vi "Project.vi"() -> ()   [LabVIEW 2016]
uses:
  <vilib>/DAQmx/read.llb/DAQmx Read (Digital Bool 1Line 1Point).vi
  <vilib>/DAQmx/write.llb/DAQmx Write (Digital Bool 1Line 1Point).vi
  <vilib>/DAQmx/create/channels.llb/DAQmx Create Channel (DO-Digital Output).vi
  <vilib>/DAQmx/create/channels.llb/DAQmx Create Channel (DI-Digital Input).vi
  <vilib>/DAQmx/miscellaneous.llb/DAQmx Fill In Error Info.vi
  <vilib>/ptbypt/NI_PtbyPt.lvlib
panel:
  in  "Emergency Stop":bool
  out "Use R2":bool
  out "Use R1":bool
  out "Register Bit #1":bool
  out "Register Bit #2":bool
  out "Output Queue Counter":dbl
  out "Rejection Pusher":bool
  out "Metal Sensor 2":bool
  out "Proximity Sensor":bool
  out "Complete or not":bool
  out "Plastic In Queue":dbl
  out "Hopper":bool
  out "Pusher":bool=TRUE
  out "Plastic or not":bool
  out "Belt 2":bool=TRUE
  out "Belt 1":bool=TRUE
  out "Stoped":bool=TRUE
  out "Started":bool=TRUE
  in  "PAUSE":bool
  in  "OFF":bool
  in  "ON":bool
  out "Rejected Pieces":dbl
  out "Completed Pieces":dbl
  out "Don't Push?":bool
  out "Is there anything there?":bool
  # "Main Control"
  # "Sorting Station"
  # "QA Sorting Station"
  # "QA Sorting Register Value"
  # "Result Counter"
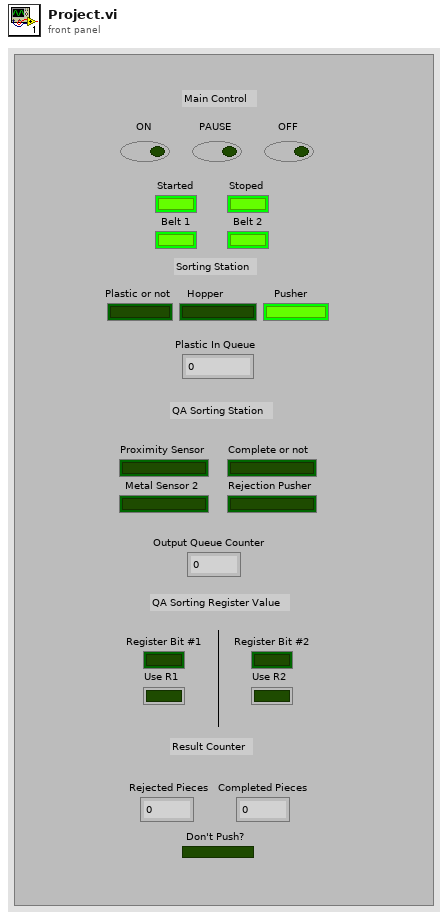
[diagram p1: front panel]
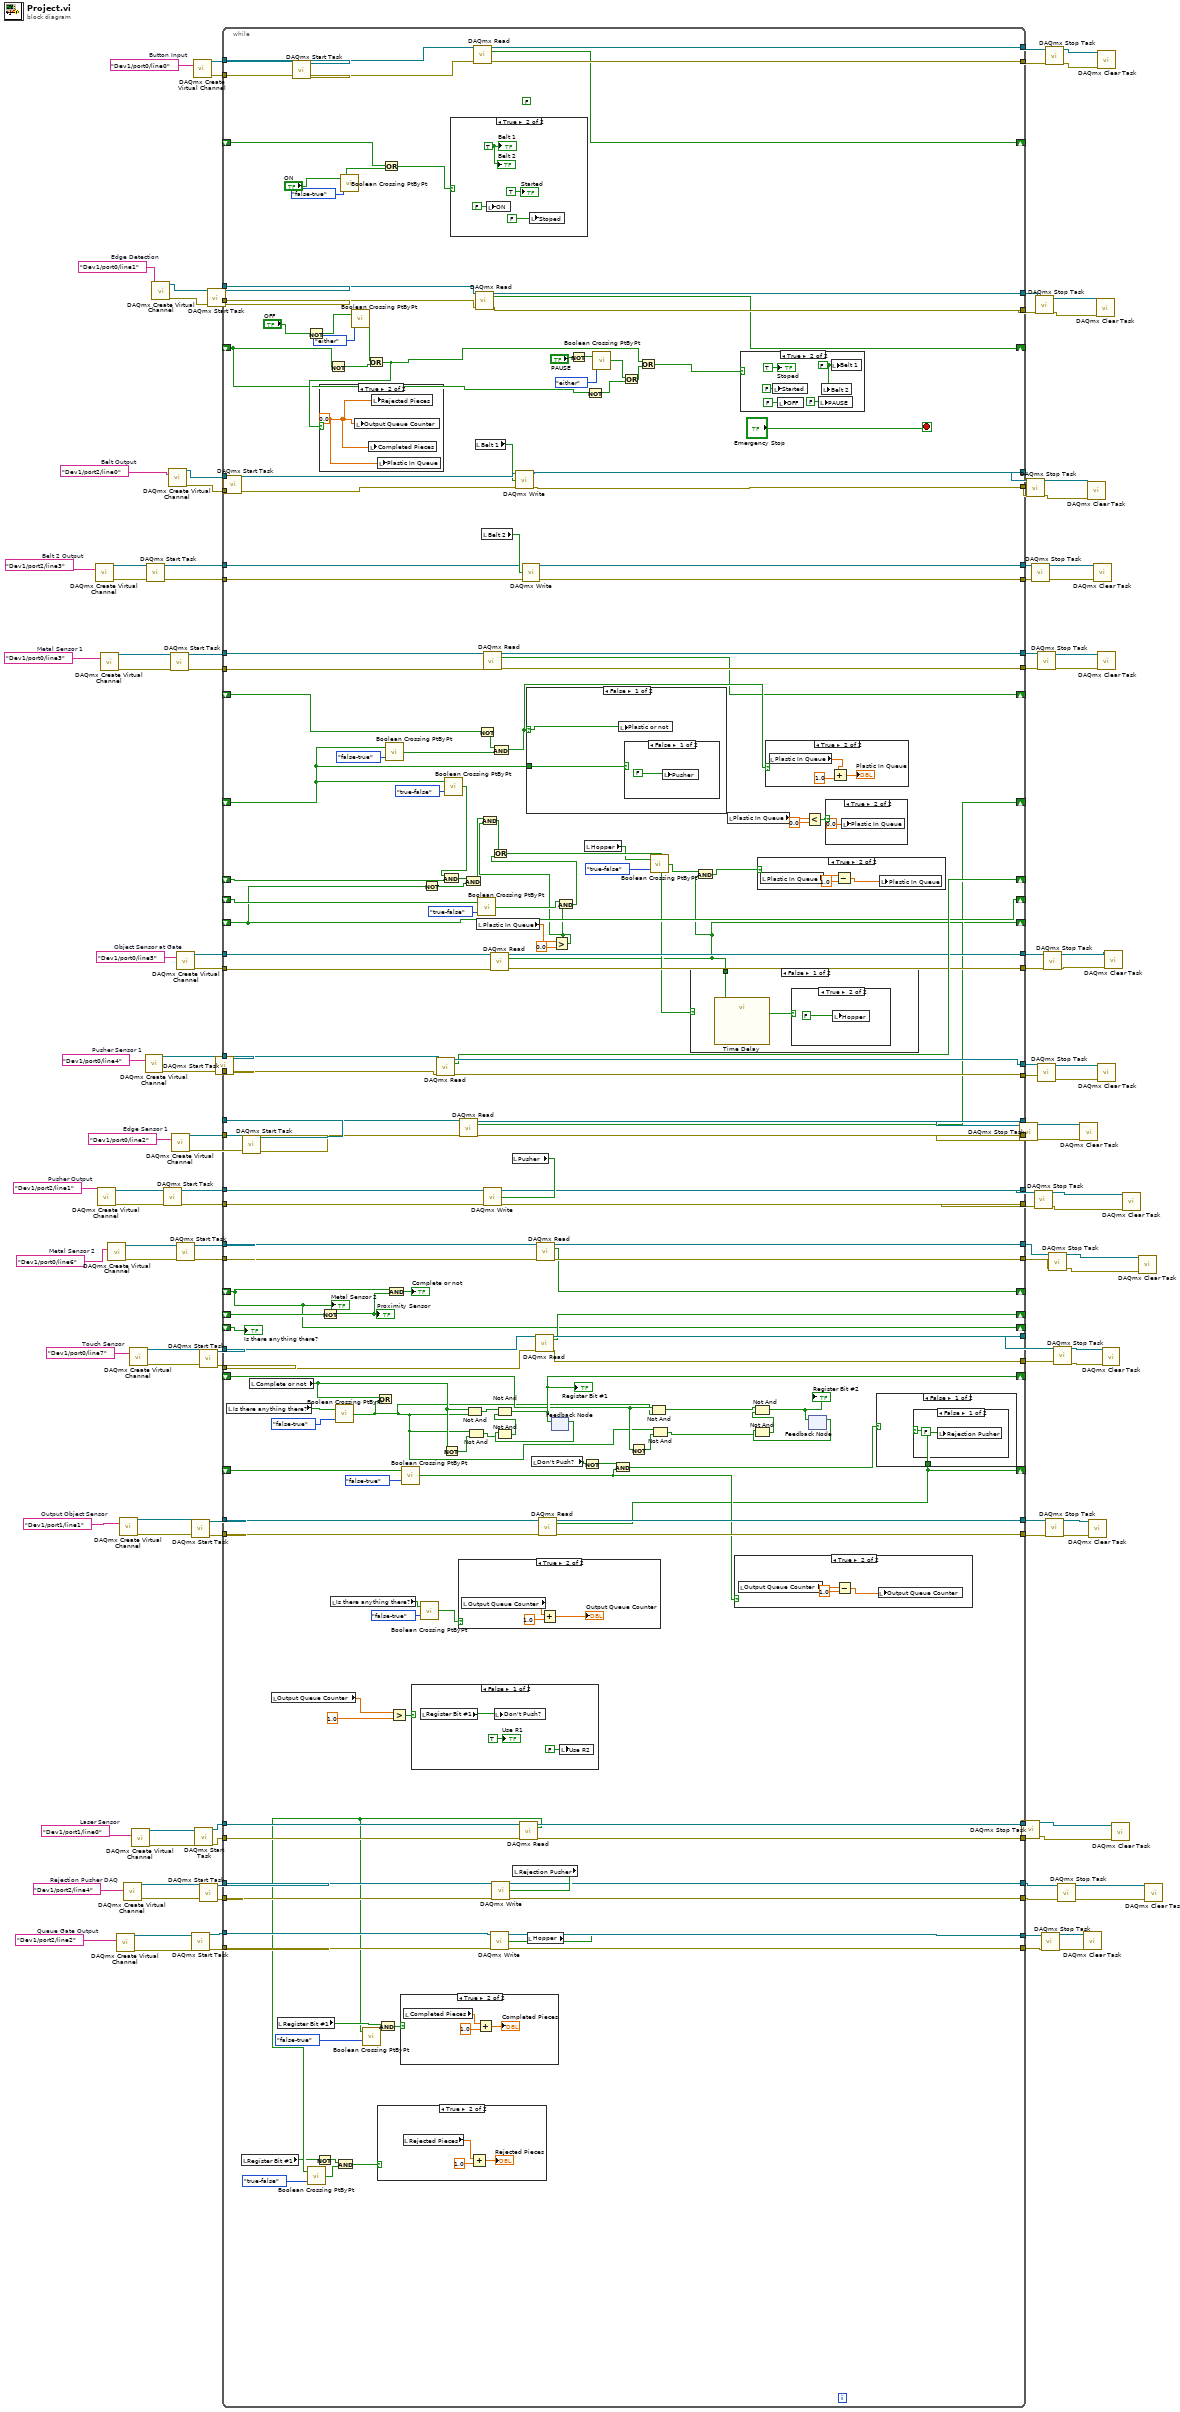
[diagram p0: block diagram]
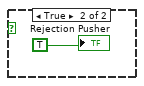
[diagram p3: hidden frame]
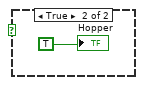
[diagram p5: hidden frame]
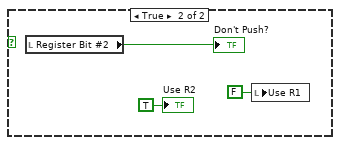
[diagram p12: hidden frame]
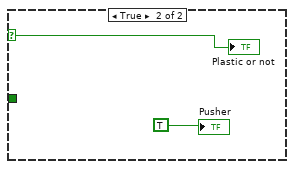
[diagram p16: hidden frame]
diagram:
  w5 = tag "Dev1/port0/line5"  # Object Sensor at Gate
  w12 = tag "Dev1/port1/line0"  # Laser Sensor
  w25 = tag "Dev1/port0/line7"  # Touch Sensor
  w28 = tag "Dev1/port1/line1"  # Output Object Sensor
  w43 = tag "Dev1/port0/line6"  # Metal Sensor 2
  w46 = tag "Dev1/port2/line4"  # Rejection Pusher DAQ
  w57 = tag "Dev1/port2/line2"  # Queue Gate Output
  w64 = tag "Dev1/port2/line3"  # Belt 2 Output
  w75 = tag "Dev1/port0/line4"  # Pusher Sensor 1
  w84 = tag "Dev1/port0/line2"  # Edge Sensor 1
  w89 = tag "Dev1/port2/line1"  # Pusher Output
  w90 = tag "Dev1/port0/line1"  # Edge Detection
  w91 = tag "Dev1/port0/line0"  # Button Input
  w92 = tag "Dev1/port0/line3"  # Metal Sensor 1
  w93 = tag "Dev1/port2/line0"  # Belt Output
  n1 = call-poly <vilib>:"DAQmx Create Virtual Channel.vi"("lines"=w64) -> ("task out"=w66:refnum<k21>, "error out"=w65:errorcluster)  [unwired: 13 in]
  n2 = call-poly <vilib>:"DAQmx Create Virtual Channel.vi"("lines"=w89) -> ("task out"=w101:refnum<k21>, "error out"=w100:errorcluster)  [unwired: 13 in]
  n3 = call-poly <vilib>:"DAQmx Create Virtual Channel.vi"("lines"=w92) -> ("task out"=w109:refnum<k21>, "error out"=w108:errorcluster)  [unwired: 13 in]
  n4 = call-poly <vilib>:"DAQmx Create Virtual Channel.vi"("lines"=w43) -> ("task out"=w45:refnum<k21>, "error out"=w44:errorcluster)  [unwired: 13 in]
  n5 = call-poly <vilib>:"DAQmx Create Virtual Channel.vi"("lines"=w57) -> ("task out"=w59:refnum<k21>, "error out"=w58:errorcluster)  [unwired: 13 in]
  n6 = call-poly <vilib>:"DAQmx Create Virtual Channel.vi"("lines"=w28) -> ("task out"=w30:refnum<k21>, "error out"=w29:errorcluster)  [unwired: 13 in]
  n7 = call-poly <vilib>:"DAQmx Create Virtual Channel.vi"("lines"=w46) -> ("task out"=w48:refnum<k21>, "error out"=w47:errorcluster)  [unwired: 13 in]
  n8 = call-poly <vilib>:"DAQmx Create Virtual Channel.vi"("lines"=w25) -> ("task out"=w27:refnum<k21>, "error out"=w26:errorcluster)  [unwired: 13 in]
  n9 = call-poly <vilib>:"DAQmx Create Virtual Channel.vi"("lines"=w12) -> ("task out"=w14:refnum<k21>, "error out"=w13:errorcluster)  [unwired: 13 in]
  n10 = call-poly <vilib>:"DAQmx Create Virtual Channel.vi"("lines"=w75) -> ("task out"=w77:refnum<k21>, "error out"=w76:errorcluster)  [unwired: 13 in]
  n11 = call <vilib>:"DAQmx Start Task.vi"("task/channels in"=w66, "error in"=w65) -> ("task out"=w63:refnum<k21>, "error out"=w62:errorcluster)  [unwired: 12 in]
  n12 = call-poly <vilib>:"DAQmx Create Virtual Channel.vi"("lines"=w90) -> ("task out"=w125:refnum<k21>, "error out"=w124:errorcluster)  [unwired: 13 in]
  n13 = call <vilib>:"DAQmx Start Task.vi"("task/channels in"=w101, "error in"=w100) -> ("task out"=w95:refnum<k21>, "error out"=w94:errorcluster)  [unwired: 12 in]
  n14 = call-poly <vilib>:"DAQmx Create Virtual Channel.vi"("lines"=w93) -> ("task out"=w113:refnum<k21>, "error out"=w112:errorcluster)  [unwired: 13 in]
  n15 = call <vilib>:"DAQmx Start Task.vi"("task/channels in"=w109, "error in"=w108) -> ("task out"=w107:refnum<k21>, "error out"=w106:errorcluster)  [unwired: 12 in]
  n16 = call-poly <vilib>:"DAQmx Create Virtual Channel.vi"("lines"=w84) -> ("task out"=w86:refnum<k21>, "error out"=w85:errorcluster)  [unwired: 13 in]
  n17 = call <vilib>:"DAQmx Start Task.vi"("task/channels in"=w45, "error in"=w44) -> ("task out"=w40:refnum<k21>, "error out"=w39:errorcluster)  [unwired: 12 in]
  n18 = call-poly <vilib>:"DAQmx Create Virtual Channel.vi"("lines"=w5) -> ("task out"=w4:refnum<k21>, "error out"=w3:errorcluster)  [unwired: 13 in]
  n19 = call <vilib>:"DAQmx Start Task.vi"("task/channels in"=w30, "error in"=w29) -> ("task out"=w24:refnum<k21>, "error out"=w23:errorcluster)  [unwired: 12 in]
  n20 = call <vilib>:"DAQmx Start Task.vi"("task/channels in"=w59, "error in"=w58) -> ("task out"=w56:refnum<k21>, "error out"=w55:errorcluster)  [unwired: 12 in]
  n21 = call-poly <vilib>:"DAQmx Create Virtual Channel.vi"("lines"=w91) -> ("task out"=w133:refnum<k21>, "error out"=w132:errorcluster)  [unwired: 13 in]
  n22 = call <vilib>:"DAQmx Start Task.vi"("task/channels in"=w14, "error in"=w13) -> ("task out"=w11:refnum<k21>, "error out"=w8:errorcluster)  [unwired: 12 in]
  n23 = call <vilib>:"DAQmx Start Task.vi"("task/channels in"=w27, "error in"=w26) -> ("task out"=w22:refnum<k21>, "error out"=w21:errorcluster)  [unwired: 12 in]
  n24 = call <vilib>:"DAQmx Start Task.vi"("task/channels in"=w48, "error in"=w47) -> ("task out"=w38:refnum<k21>, "error out"=w37:errorcluster)  [unwired: 12 in]
  n25 = call <vilib>:"DAQmx Start Task.vi"("task/channels in"=w125, "error in"=w124) -> ("task out"=w122:refnum<k21>, "error out"=w123:errorcluster)  [unwired: 12 in]
  n26 = call <vilib>:"DAQmx Start Task.vi"("task/channels in"=w77, "error in"=w76) -> ("task out"=w74:refnum<k21>, "error out"=w73:errorcluster)  [unwired: 12 in]
  n27 = call <vilib>:"DAQmx Start Task.vi"("task/channels in"=w113, "error in"=w112) -> ("task out"=w111:refnum<k21>, "error out"=w110:errorcluster)  [unwired: 12 in]
  n28 = call <vilib>:"DAQmx Start Task.vi"("task/channels in"=w86, "error in"=w85) -> ("task out"=w83:refnum<k21>, "error out"=w82:errorcluster)  [unwired: 12 in]
  n29 = call <vilib>:"DAQmx Start Task.vi"("task/channels in"=w133, "error in"=w132) -> ("task out"=w131:refnum<k21>, "error out"=w130:errorcluster)  [unwired: 12 in]
  n30 = while {
    tunnel: w131 -> [w300]
    tunnel: w130 -> [w299]
    tunnel: [w298] -> w129
    tunnel: [w297] -> w128
    shift-right: [w295] -> _
    shift-left: _ -> [w229]
    tunnel: w123 -> [w294]
    tunnel: w122 -> [w293]
    tunnel: [w292] -> w121
    tunnel: [w291] -> w118
    shift-right: [w290] -> _
    shift-left: _ -> [w167]
    tunnel: [w289] -> w115
    tunnel: [w286] -> w114
    tunnel: w111 -> [w288]
    tunnel: w110 -> [w287]
    tunnel: w107 -> [w284]
    tunnel: w106 -> [w283]
    tunnel: [w282] -> w103
    tunnel: [w281] -> w102
    shift-right: [w139] -> _
    shift-left: _ -> [w138]
    tunnel: [w279] -> w97
    tunnel: [w278] -> w96
    tunnel: w95 -> [w277]
    tunnel: w94 -> [w276]
    tunnel: w83 -> [w275]
    tunnel: w82 -> [w274]
    tunnel: [w273] -> w81
    tunnel: [w272] -> w80
    shift-right: [w141] -> _
    shift-left: _ -> [w134]
    tunnel: w74 -> [w270]
    tunnel: w73 -> [w269]
    tunnel: [w268] -> w72
    tunnel: [w267] -> w71
    tunnel: [w264] -> w68
    tunnel: [w263] -> w67
    tunnel: w63 -> [w262]
    tunnel: w62 -> [w261]
    tunnel: w56 -> [w260]
    tunnel: w55 -> [w259]
    tunnel: [w258] -> w54
    tunnel: [w257] -> w53
    shift-right: [w255] -> _
    shift-left: _ -> [w254]
    tunnel: [w250] -> w42
    tunnel: [w249] -> w41
    tunnel: w40 -> [w248]
    tunnel: w39 -> [w247]
    tunnel: w38 -> [w246]
    tunnel: w37 -> [w245]
    tunnel: [w244] -> w36
    tunnel: [w243] -> w35
    shift-right: [w242] -> _
    shift-left: _ -> [w195]
    tunnel: w24 -> [w241]
    tunnel: w23 -> [w240]
    tunnel: w22 -> [w239]
    tunnel: w21 -> [w238]
    tunnel: [w237] -> w20
    tunnel: [w236] -> w19
    tunnel: [w235] -> w18
    tunnel: [w234] -> w17
    shift-right: [w142] -> _
    shift-left: _ -> [w217]
    shift-right: [w233] -> _
    shift-left: _ -> [w232]
    shift-right: [w195] -> _
    shift-left: _ -> [w219]
    tunnel: w11 -> [w215]
    tunnel: [w214] -> w10
    tunnel: [w213] -> w9
    tunnel: w8 -> [w212]
    shift-right: [w197] -> _
    shift-left: _ -> [w196]
    tunnel: w4 -> [w166]
    tunnel: w3 -> [w165]
    tunnel: [w164] -> w2
    tunnel: [w163] -> w1
    shift-right: [w136] -> _
    shift-left: _ -> [w158]
    shift-right: [w158] -> _
    shift-left: _ -> [w161]
    stop <- "Emergency Stop" stop-if-true
    (unwired) FALSE ("Boolean")
    n31 = local read "Is there anything there?"() -> (w220:bool)
    n32 = local read "Register Bit #1"() -> (w176:bool)
    n33 = local read "Complete or not"() -> (w194:bool)
    n34 = local read "Output Queue Counter"() -> (w205:dbl)
    n35 = local read "Register Bit #1"() -> (w183:bool)
    n36 = Not(x="OFF") -> (.not. x?=w189:bool)
    n37 = Not(x=w176) -> (.not. x?=w177:bool)
    n38 = Not(x=w232) -> (.not. x?=w227:bool)
    "Proximity Sensor" <- w227
    n39 = Not(x=w167) -> (.not. x?=w228:bool)
    n40 = local read "Is there anything there?"() -> (w209:bool)
    n41 = call <vilib>:"Boolean Crossing PtByPt.vi"("direction"=enum16{"either", "false-true", "true-false"}."false-true", "input"=w220) -> ("crossing"=w193:bool)  [unwired: 1 in]
    n42 = call <vilib>:"Boolean Crossing PtByPt.vi"("direction"=enum16{"either", "false-true", "true-false"}."false-true", "input"="ON") -> ("crossing"=w192:bool)  [unwired: 1 in]
    n43 = call <vilib>:"Boolean Crossing PtByPt.vi"("direction"=enum16{"either", "false-true", "true-false"}."either", "input"=w189) -> ("crossing"=w190:bool)  [unwired: 1 in]
    n44 = Or(x=w190, y=w228) -> (x .or. y?=w168:bool)
    n45 = case shown="True" w168 {
      frame False {
      }
      frame True {
        w314 = 0.0 ("Completed Piece")
        n46 = local write "Output Queue Counter"(w314) -> ()
        n47 = local write "Completed Pieces"(w314) -> ()
        n48 = local write "Rejected Pieces"(w314) -> ()
        n49 = local write "Plastic In Queue"(w314) -> ()
      }
    }
    n50 = Or(x=w194, y=w193) -> ()  [unwired: 1 out]
    n51 = Or(x=w229, y=w192) -> (x .or. y?=w230:bool)
    n52 = call <vilib>:"Boolean Crossing PtByPt.vi"("direction"=enum16{"either", "false-true", "true-false"}."false-true", "input"=w134) -> ("crossing"=w256:bool)  [unwired: 1 in]
    n53 = And(x=w195, y=w227) -> (x .and. y?=→"Complete or not":bool)
    n54 = Greater?(x=w205, y=1.0) -> (0:w204:bool)
    n55 = call <vilib>:"Boolean Crossing PtByPt.vi"("direction"=enum16{"either", "false-true", "true-false"}."false-true", "input"=w217) -> ("crossing"=w207:bool)  [unwired: 1 in]
    n56 = case shown="False" w204 {
      frame False {
        n57 = local read "Register Bit #1"() -> (w323:bool)
        n58 = local write "Don't Push?"(w323) -> ()
        n59 = local write "Use R2"(FALSE ("Use R2")) -> ()
        "Use R1" <- TRUE ("Use R1")
      }
      frame True {
        n60 = local read "Register Bit #2"() -> (→"Don't Push?":bool)
        n61 = local write "Use R1"(FALSE ("Use R1")) -> ()
        "Use R2" <- TRUE ("Use R2")
      }
    }
    n62 = call <vilib>:"Boolean Crossing PtByPt.vi"("direction"=enum16{"either", "false-true", "true-false"}."false-true", "input"=w209) -> ("crossing"=w210:bool)  [unwired: 1 in]
    n63 = Not(x=w158) -> (.not. x?=w159:bool)
    n64 = call-poly <vilib>:"DAQmx Read.vi"("task/channels in"=w270, "error in"=w269) -> ("task out"=w267:refnum<k21>, "data"=w255:bool, "error out"=w268:errorcluster)  [unwired: 11 in]
    n65 = Not(x=w194) -> (.not. x?=w222:bool)
    n66 = call <vilib>:"Boolean Crossing PtByPt.vi"("direction"=enum16{"either", "false-true", "true-false"}."true-false", "input"=w134) -> ("crossing"=w252:bool)  [unwired: 1 in]
    n67 = And(x=w252, y=w254) -> (x .and. y?=w160:bool)
    n68 = case shown="True" w230 {
      frame False {
      }
      frame True {
        w344 = TRUE
        n69 = local write "ON"(FALSE ("ON")) -> ()
        n70 = local write "Stoped"(FALSE) -> ()
        "Started" <- TRUE ("Boolean")
        "Belt 1" <- w344
        "Belt 2" <- w344
      }
    }
    n71 = case shown="True" w210 {
      frame False {
      }
      frame True {
        n72 = local read "Output Queue Counter"() -> (w330:dbl)
        n73 = Add(x=w330, y=1.0) -> (x+y=→"Output Queue Counter":dbl)
      }
    }
    n74 = call-poly <vilib>:"DAQmx Read.vi"("task/channels in"=w275, "error in"=w274) -> ("task out"=w272:refnum<k21>, "data"=w141:bool, "error out"=w273:errorcluster)  [unwired: 11 in]
    n75 = And(x=w160, y=w159) -> (x .and. y?=w152:bool)
    n76 = Not And(1:w193, 2:w194) -> (0:w223:bool)
    n77 = Not And(1:w222, 2:w193) -> (0:w224:bool)
    n78 = call-poly <vilib>:"DAQmx Read.vi"("task/channels in"=w300, "error in"=w299) -> ("task out"=w298:refnum<k21>, "data"=w295:bool, "error out"=w297:errorcluster)  [unwired: 11 in]
    n79 = call-poly <vilib>:"DAQmx Read.vi"("task/channels in"=w293, "error in"=w294) -> ("task out"=w292:refnum<k21>, "data"=w290:bool, "error out"=w291:errorcluster)  [unwired: 11 in]
    n80 = local read "Belt 1"() -> (w285:bool)
    n81 = local read "Plastic In Queue"() -> (w156:dbl)
    n82 = call <vilib>:"Boolean Crossing PtByPt.vi"("direction"=enum16{"either", "false-true", "true-false"}."true-false", "input"=w161) -> ("crossing"=w154:bool)  [unwired: 1 in]
    n83 = Not(x=w138) -> (.not. x?=w271:bool)
    n84 = local read "Belt 2"() -> (w265:bool)
    n85 = call-poly <vilib>:"DAQmx Read.vi"("task/channels in"=w284, "error in"=w283) -> ("task out"=w282:refnum<k21>, "data"=w139:bool, "error out"=w281:errorcluster)  [unwired: 11 in]
    n86 = call-poly <vilib>:"DAQmx Read.vi"("task/channels in"=w166, "error in"=w165) -> ("task out"=w164:refnum<k21>, "data"=w136:bool, "error out"=w163:errorcluster)  [unwired: 11 in]
    n87 = And(x=w271, y=w256) -> (x .and. y?=w157:bool)
    n88 = local read "Pusher"() -> (w280:bool)
    n89 = call-poly <vilib>:"DAQmx Write.vi"("task/channels in"=w277, "data"=w280, "error in"=w276) -> ("task out"=w279:refnum<k21>, "error out"=w278:errorcluster)  [unwired: 10 in, 1 out]
    n90 = local read "Rejection Pusher"() -> (w251:bool)
    n91 = call-poly <vilib>:"DAQmx Write.vi"("task/channels in"=w246, "data"=w251, "error in"=w245) -> ("task out"=w244:refnum<k21>, "error out"=w243:errorcluster)  [unwired: 10 in, 1 out]
    n92 = call-poly <vilib>:"DAQmx Write.vi"("task/channels in"=w288, "data"=w285, "error in"=w287) -> ("task out"=w289:refnum<k21>, "error out"=w286:errorcluster)  [unwired: 10 in, 1 out]
    n93 = call-poly <vilib>:"DAQmx Read.vi"("task/channels in"=w215, "error in"=w212) -> ("task out"=w214:refnum<k21>, "data"=w180:bool, "error out"=w213:errorcluster)  [unwired: 11 in]
    n94 = call <vilib>:"Boolean Crossing PtByPt.vi"("direction"=enum16{"either", "false-true", "true-false"}."true-false", "input"=w180) -> ("crossing"=w178:bool)  [unwired: 1 in]
    n95 = And(x=w177, y=w178) -> (x .and. y?=w179:bool)
    n96 = call <vilib>:"Boolean Crossing PtByPt.vi"("direction"=enum16{"either", "false-true", "true-false"}."false-true", "input"=w180) -> ("crossing"=w182:bool)  [unwired: 1 in]
    n97 = case shown="True" w179 {
      frame False {
      }
      frame True {
        n98 = local read "Rejected Pieces"() -> (w316:dbl)
        n99 = Add(x=w316, y=1.0) -> (x+y=→"Rejected Pieces":dbl)
      }
    }
    n100 = And(x=w183, y=w182) -> (x .and. y?=w181:bool)
    n101 = case shown="True" w181 {
      frame False {
      }
      frame True {
        n102 = local read "Completed Pieces"() -> (w318:dbl)
        n103 = Add(x=w318, y=1.0) -> (x+y=→"Completed Pieces":dbl)
      }
    }
    n104 = call-poly <vilib>:"DAQmx Write.vi"("task/channels in"=w262, "data"=w265, "error in"=w261) -> ("task out"=w264:refnum<k21>, "error out"=w263:errorcluster)  [unwired: 10 in, 1 out]
    n105 = case shown="False" w157 {
      selector: w157 -> [w334 w337]
      tunnel: w134 -> [w333 _]
      frame False {
        n106 = local write "Plastic or not"(w334) -> ()
        n107 = case shown="False" w333 {
          frame False {
            n108 = local write "Pusher"(FALSE) -> ()
          }
          frame True {
          }
        }
      }
      frame True {
        "Plastic or not" <- w337
        "Pusher" <- TRUE
      }
    }
    n109 = local read "Hopper"() -> (w231:bool)
    n110 = call-poly <vilib>:"DAQmx Write.vi"("task/channels in"=w260, "data"=w231, "error in"=w259) -> ("task out"=w258:refnum<k21>, "error out"=w257:errorcluster)  [unwired: 10 in, 1 out]
    n111 = local read "Don't Push?"() -> (w211:bool)
    n112 = call-poly <vilib>:"DAQmx Read.vi"("task/channels in"=w239, "error in"=w238) -> ("task out"=w234:refnum<k21>, "data"=w233:bool, "error out"=w235:errorcluster)  [unwired: 11 in]
    n113 = call-poly <vilib>:"DAQmx Read.vi"("task/channels in"=w248, "error in"=w247) -> ("task out"=w250:refnum<k21>, "data"=w242:bool, "error out"=w249:errorcluster)  [unwired: 11 in]
    n114 = call-poly <vilib>:"DAQmx Read.vi"("task/channels in"=w241, "error in"=w240) -> ("task out"=w237:refnum<k21>, "data"=w142:bool, "error out"=w236:errorcluster)  [unwired: 11 in]
    n115 = feedback #1() -> (w225:bool)  [unwired: 1 in]
    n116 = Not And(1:w224, 2:w225) -> (0:w226:bool)
    n117 = Not And(1:w226, 2:w223) -> (0:w197:bool)
    "Register Bit #1" <- w197
    n118 = feedback-in #1(w197) -> ()
    n119 = Greater?(x=w156, y=0.0) -> (0:w151:bool)
    n120 = And(x=w152, y=w151) -> (x .and. y?=w146:bool)
    n121 = And(x=w154, y=w151) -> (x .and. y?=w145:bool)
    n122 = Or(x=w146, y=w145) -> (x .or. y?=w144:bool)
    n123 = Not(x="PAUSE") -> (.not. x?=w173:bool)
    n124 = Not(x=w211) -> (.not. x?=w218:bool)
    n125 = local read "Hopper"() -> (w140:bool)
    n126 = Not(x=w167) -> (.not. x?=w175:bool)
    n127 = call <vilib>:"Boolean Crossing PtByPt.vi"("direction"=enum16{"either", "false-true", "true-false"}."either", "input"=w173) -> ("crossing"=w174:bool)  [unwired: 1 in]
    n128 = And(x=w218, y=w207) -> (x .and. y?=w143:bool)
    n129 = Or(x=w174, y=w175) -> (x .or. y?=w169:bool)
    n130 = Not(x=w196) -> (.not. x?=w199:bool)
    n131 = Or(x=w168, y=w169) -> (x .or. y?=w170:bool)
    n132 = call <vilib>:"Boolean Crossing PtByPt.vi"("direction"=enum16{"either", "false-true", "true-false"}."true-false", "input"=w140) -> ("crossing"=w137:bool)  [unwired: 1 in]
    n133 = Not And(1:w193, 2:w196) -> (0:w200:bool)
    n134 = Not And(1:w199, 2:w193) -> (0:w201:bool)
    n135 = case shown="False" w144 {
      tunnel: w136 -> [w304 _]
      frame False {
        n136 = call "Time Delay"() -> ()  [unwired: 11 in, 1 out]
        n137 = case shown="True" w304 {
          frame False {
          }
          frame True {
            n138 = local write "Hopper"(FALSE) -> ()
          }
        }
      }
      frame True {
        "Hopper" <- TRUE
      }
    }
    n139 = And(x=w137, y=w136) -> (x .and. y?=w135:bool)
    n140 = local read "Plastic In Queue"() -> (w150:dbl)
    n141 = case shown="True" w207 {
      frame False {
      }
      frame True {
        n142 = local read "Output Queue Counter"() -> (w329:dbl)
        n143 = Subtract(x=w329, y=1.0) -> (x-y=w327:dbl)
        n144 = local write "Output Queue Counter"(w327) -> ()
      }
    }
    n145 = case shown="True" w170 {
      frame False {
      }
      frame True {
        w340 = FALSE
        n146 = local write "Started"(FALSE ("Stop")) -> ()
        n147 = local write "OFF"(FALSE ("OFF")) -> ()
        n148 = local write "PAUSE"(FALSE ("Pause")) -> ()
        n149 = local write "Belt 2"(w340) -> ()
        n150 = local write "Belt 1"(w340) -> ()
        "Stoped" <- TRUE
      }
    }
    n151 = case shown="True" w135 {
      frame False {
      }
      frame True {
        n152 = local read "Plastic In Queue"() -> (w309:dbl)
        n153 = Subtract(x=w309, y=1.0) -> (x-y=w310:dbl)
        n154 = local write "Plastic In Queue"(w310) -> ()
      }
    }
    n155 = case shown="True" w157 {
      frame False {
      }
      frame True {
        n156 = local read "Plastic In Queue"() -> (w311:dbl)
        n157 = Add(x=w311, y=1.0) -> (x+y=→"Plastic In Queue":dbl)
      }
    }
    n158 = Less?(x=w150, y=0.0) -> (x < y?=w148:bool)
    n159 = feedback #2() -> (w202:bool)  [unwired: 1 in]
    n160 = Not And(1:w201, 2:w202) -> (0:w203:bool)
    n161 = Not And(1:w203, 2:w200) -> (0:w198:bool)
    "Register Bit #2" <- w198
    n162 = feedback-in #2(w198) -> ()
    n163 = case shown="True" w148 {
      frame False {
      }
      frame True {
        n164 = local write "Plastic In Queue"(0.0 ("Plastic In Queue")) -> ()
      }
    }
    n165 = case shown="False" w143 {
      tunnel: w142 -> [w301 _]
      frame False {
        n166 = case shown="False" w301 {
          frame False {
            n167 = local write "Rejection Pusher"(FALSE) -> ()
          }
          frame True {
          }
        }
      }
      frame True {
        "Rejection Pusher" <- TRUE
      }
    }
    "Metal Sensor 2" <- w195
    "Is there anything there?" <- w219
  }
  n168 = call <vilib>:"DAQmx Stop Task.vi"("task/channels in"=w80, "error in"=w81) -> ("task out"=w88:refnum<k21>, "error out"=w87:errorcluster)  [unwired: 12 in]
  n169 = call <vilib>:"DAQmx Stop Task.vi"("task/channels in"=w10, "error in"=w9) -> ("task out"=w16:refnum<k21>, "error out"=w15:errorcluster)  [unwired: 12 in]
  n170 = call <vilib>:"DAQmx Stop Task.vi"("task/channels in"=w115, "error in"=w114) -> ("task out"=w117:refnum<k21>, "error out"=w116:errorcluster)  [unwired: 12 in]
  n171 = call <vilib>:"DAQmx Stop Task.vi"("task/channels in"=w68, "error in"=w67) -> ("task out"=w70:refnum<k21>, "error out"=w69:errorcluster)  [unwired: 12 in]
  n172 = call <vilib>:"DAQmx Stop Task.vi"("task/channels in"=w97, "error in"=w96) -> ("task out"=w99:refnum<k21>, "error out"=w98:errorcluster)  [unwired: 12 in]
  n173 = call <vilib>:"DAQmx Stop Task.vi"("task/channels in"=w121, "error in"=w118) -> ("task out"=w120:refnum<k21>, "error out"=w119:errorcluster)  [unwired: 12 in]
  n174 = call <vilib>:"DAQmx Stop Task.vi"("task/channels in"=w103, "error in"=w102) -> ("task out"=w105:refnum<k21>, "error out"=w104:errorcluster)  [unwired: 12 in]
  n175 = call <vilib>:"DAQmx Stop Task.vi"("task/channels in"=w71, "error in"=w72) -> ("task out"=w79:refnum<k21>, "error out"=w78:errorcluster)  [unwired: 12 in]
  n176 = call <vilib>:"DAQmx Stop Task.vi"("task/channels in"=w54, "error in"=w53) -> ("task out"=w61:refnum<k21>, "error out"=w60:errorcluster)  [unwired: 12 in]
  n177 = call <vilib>:"DAQmx Stop Task.vi"("task/channels in"=w2, "error in"=w1) -> ("task out"=w7:refnum<k21>, "error out"=w6:errorcluster)  [unwired: 12 in]
  n178 = call <vilib>:"DAQmx Stop Task.vi"("task/channels in"=w20, "error in"=w19) -> ("task out"=w34:refnum<k21>, "error out"=w33:errorcluster)  [unwired: 12 in]
  n179 = call <vilib>:"DAQmx Stop Task.vi"("task/channels in"=w129, "error in"=w128) -> ("task out"=w126:refnum<k21>, "error out"=w127:errorcluster)  [unwired: 12 in]
  n180 = call <vilib>:"DAQmx Stop Task.vi"("task/channels in"=w42, "error in"=w41) -> ("task out"=w50:refnum<k21>, "error out"=w49:errorcluster)  [unwired: 12 in]
  n181 = call <vilib>:"DAQmx Stop Task.vi"("task/channels in"=w17, "error in"=w18) -> ("task out"=w32:refnum<k21>, "error out"=w31:errorcluster)  [unwired: 12 in]
  n182 = call <vilib>:"DAQmx Stop Task.vi"("task/channels in"=w36, "error in"=w35) -> ("task out"=w52:refnum<k21>, "error out"=w51:errorcluster)  [unwired: 12 in]
  n183 = call <vilib>:"DAQmx Clear Task.vi"("task in"=w88, "error in"=w87) -> ()  [unwired: 13 in, 1 out]
  n184 = call <vilib>:"DAQmx Clear Task.vi"("task in"=w61, "error in"=w60) -> ()  [unwired: 13 in, 1 out]
  n185 = call <vilib>:"DAQmx Clear Task.vi"("task in"=w117, "error in"=w116) -> ()  [unwired: 13 in, 1 out]
  n186 = call <vilib>:"DAQmx Clear Task.vi"("task in"=w34, "error in"=w33) -> ()  [unwired: 13 in, 1 out]
  n187 = call <vilib>:"DAQmx Clear Task.vi"("task in"=w70, "error in"=w69) -> ()  [unwired: 13 in, 1 out]
  n188 = call <vilib>:"DAQmx Clear Task.vi"("task in"=w120, "error in"=w119) -> ()  [unwired: 13 in, 1 out]
  n189 = call <vilib>:"DAQmx Clear Task.vi"("task in"=w126, "error in"=w127) -> ()  [unwired: 13 in, 1 out]
  n190 = call <vilib>:"DAQmx Clear Task.vi"("task in"=w105, "error in"=w104) -> ()  [unwired: 13 in, 1 out]
  n191 = call <vilib>:"DAQmx Clear Task.vi"("task in"=w79, "error in"=w78) -> ()  [unwired: 13 in, 1 out]
  n192 = call <vilib>:"DAQmx Clear Task.vi"("task in"=w32, "error in"=w31) -> ()  [unwired: 13 in, 1 out]
  n193 = call <vilib>:"DAQmx Clear Task.vi"("task in"=w7, "error in"=w6) -> ()  [unwired: 13 in, 1 out]
  n194 = call <vilib>:"DAQmx Clear Task.vi"("task in"=w16, "error in"=w15) -> ()  [unwired: 13 in, 1 out]
  n195 = call <vilib>:"DAQmx Clear Task.vi"("task in"=w99, "error in"=w98) -> ()  [unwired: 13 in, 1 out]
  n196 = call <vilib>:"DAQmx Clear Task.vi"("task in"=w50, "error in"=w49) -> ()  [unwired: 13 in, 1 out]
  n197 = call <vilib>:"DAQmx Clear Task.vi"("task in"=w52, "error in"=w51) -> ()  [unwired: 13 in, 1 out]
